vi "REQ Initialize DI.vi"(6 "wait for reply (T)":bool=TRUE, 8 "error in":errorcluster, 10 "Boolean":bool, 11 "DI Channel Setting":T1) -> (0 "error out":errorcluster, 1 "timed out?":bool, 3 "Connect?":bool)   [LabVIEW 2016, in "DAQ Hardware.lvlib"]
doc: "_____\nCreated using DQMH Event Scripter 6.1.0.128."
uses:
  DAQ Hardware.lvlib
  DI Channel Setting.ctl
  REQ Initialize DI Argument--cluster.ctl
  REQ Initialize DI (Reply Payload)--cluster.ctl
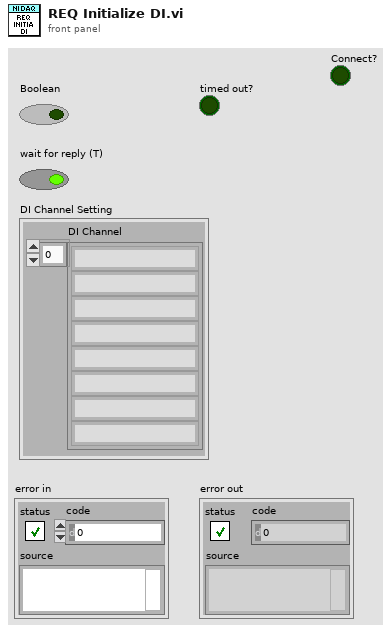
[diagram p1: front panel]
types:
  T1 = typedef "DAQ Hardware.lvlib/DI Channel Setting.ctl" = cluster{"DI Channel":string[]}
  T2 = typedef "DAQ Hardware.lvlib/REQ Initialize DI Argument--cluster.ctl" = cluster{"Boolean":bool, "Wait Notifier":refnum<notifier>, "wait for reply":bool, "DI Channel Setting":T1}
  T3 = typedef "DAQ Hardware.lvlib/Request Events--cluster.ctl" = cluster{"Stop Module":refnum<user-event>, "Show Panel":refnum<user-event>, "Hide Panel":refnum<user-event>, "Get Module Execution Status":refnum<user-event>, "Show Diagram":refnum<user-event>, "REQ Initialize AI":refnum<user-event>, "REQ Initialize AO":refnum<user-event>, "REQ Initialize DI":refnum<user-event>, "REQ Initialize DO":refnum<user-event>, "REQ Write DO":refnum<user-event>, "REQ Acquire AI":refnum<user-event>, "REQ Close Ref":refnum<user-event>, "REQ Write AO":refnum<user-event>, "REQ Update Sample Rate":refnum<user-event>, "REQ Acquire DI":refnum<user-event>, "REQ Wakeup_Helper_loop_AI":refnum<user-event>, "REQ Retry AI":refnum<user-event>, "REQ Wakeup_helper_loop_DI":refnum<user-event>, "REQ Retry DI":refnum<user-event>, "Write AO Data":refnum<user-event>, "REQ Log Data":refnum<user-event>}
  T4 = typedef "DAQ Hardware.lvlib/REQ Initialize DI (Reply Payload)--cluster.ctl" = cluster{"error":errorcluster, "Connect?":bool}
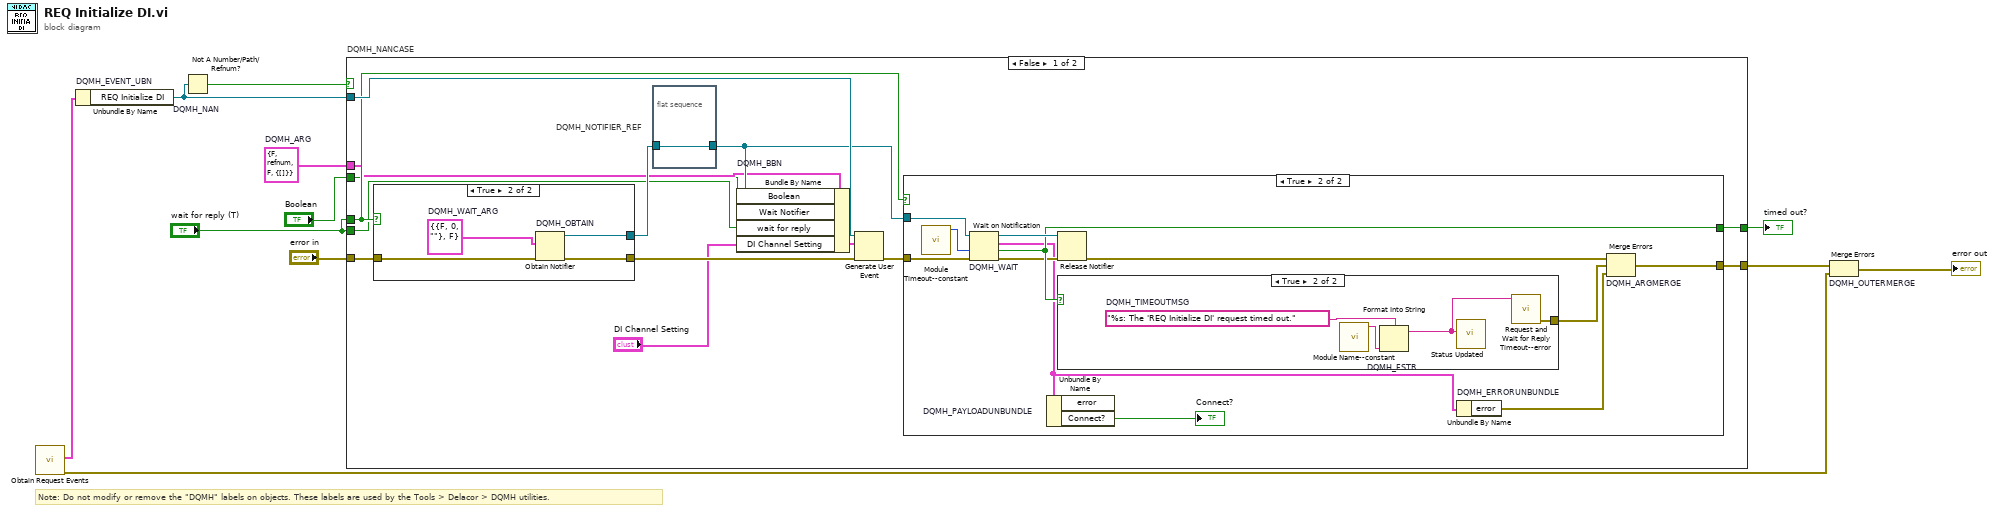
[diagram p0: block diagram]
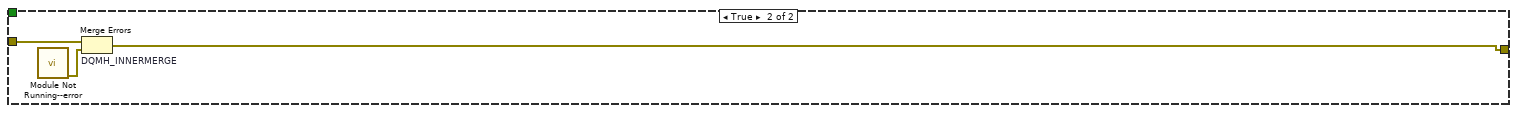
[diagram p5: hidden frame]
diagram:
  w5 = T2 {"Boolean"=FALSE, "Wait Notifier"=refnum, "wait for reply"=FALSE, "DI Channel Setting"={"DI Channel"=[]}}  # DQMH_ARG
  # "Note: Do not modify or remove the \"DQMH\" labels on objects. These labels are used by the Tools > Delacor > DQMH utilities."
  n1 = call "Obtain Request Events.vi"() -> ("error out"=w2:errorcluster, "DAQ Hardware Request Events"=w1:T3)  [unwired: 10 in]
  n2 = Unbundle By Name "DQMH_EVENT_UBN"(w1) -> ("REQ Initialize DI"=w6:refnum<user-event>)
  n3 = Not A Number/Path/Refnum? "DQMH_NAN"(number/path/refnum=w6) -> (NaN/Path/Refnum?=w7:bool)
  n4 = case "DQMH_NANCASE" shown="False" w7 {
    tunnel: "error in" -> [w25 w51]
    tunnel: w6 -> [w23 _]
    tunnel: [w20 w50] -> w8
    tunnel: [w21 _] -> w10
    tunnel: "wait for reply (T)" -> [w18 _]
    tunnel: w5 -> [w15 _]
    tunnel: "Boolean" -> [w14 _]
    tunnel: "wait for reply (T)" -> [w13 _]
    frame False {
      n5 = case shown="True" w18 {
        tunnel: w25 -> [w44 w48]
        tunnel: [w44 w47] -> w22
        tunnel: [_ w45] -> w17
        frame False {
        }
        frame True {
          w46 = T4 {"error"={"status"=FALSE, "code"=0, "source"=""}, "Connect?"=FALSE}  # DQMH_WAIT_ARG
          n6 = Obtain Notifier "DQMH_OBTAIN"(notification data type=w46, error in (no error)=w48) -> (notifier out=w45:refnum<notifier>, error out=w47:errorcluster)  [unwired: 2 in, 1 out]
        }
      }
      n7 = flat-sequence "DQMH_NOTIFIER_REF" {
        tunnel: w17 -> [w26]
        tunnel: [w26] -> w16
        frame #0 {
        }
      }
      n8 = Bundle By Name "DQMH_BBN"(cluster=w15, "Boolean"=w14, "Wait Notifier"=w16, "wait for reply"=w13, "DI Channel Setting"="DI Channel Setting") -> (w19:T2)
      n9 = Generate User Event(user event=w23, event data cluster=w19, error in=w22) -> (error out=w24:errorcluster)  [unwired: 1 in, 1 out]
      n10 = case shown="True" w18 {
        tunnel: w24 -> [w27 w39]
        tunnel: w16 -> [_ w38]
        tunnel: [_ w36] -> w21
        tunnel: [w27 w35] -> w20
        frame False {
        }
        frame True {
          n11 = call "Module Timeout--constant.vi"() -> ("Module Timeout"=w29:i32)  [unwired: 11 in]
          n12 = Wait on Notification "DQMH_WAIT"(notifier=w38, timeout in ms (-1)=w29, error in (no error)=w39) -> (notifier out=w37:refnum<notifier>, notification=w30:T4, timed out?=w36:bool, error out=w34:errorcluster)  [unwired: 1 in]
          n13 = Unbundle By Name "DQMH_PAYLOADUNBUNDLE"(w30) -> ("Connect?"=→"Connect?":bool)  [unwired: 1 out]
          n14 = Release Notifier(notifier=w37, error in (no error)=w34) -> (error out=w33:errorcluster)  [unwired: 1 in, 2 out]
          n15 = case shown="True" w36 {
            tunnel: [_ w41] -> w31
            frame False {
            }
            frame True {
              w43 = "%s: The 'REQ Initialize DI' request timed out."  # DQMH_TIMEOUTMSG
              n16 = call "Module Name--constant.vi"() -> ("Module Name"=w40:string)  [unwired: 11 in]
              n17 = Format Into String "DQMH_FSTR"(format string=w43, w40) -> (resulting string=w42:string)  [unwired: 2 in, 1 out]
              n18 = call "Status Updated.vi"("Status"=w42) -> ()  [unwired: 10 in, 1 out]
              n19 = call "Request and Wait for Reply Timeout--error.vi"("Error Message"=w42) -> ("error out"=w41:errorcluster)  [unwired: 10 in]
            }
          }
          n20 = Unbundle By Name "DQMH_ERRORUNBUNDLE"(w30) -> ("error"=w32:errorcluster)
          n21 = Merge Errors "DQMH_ARGMERGE"(w33, w31, w32) -> (w35:errorcluster)
        }
      }
    }
    frame True {
      n22 = call "Module Not Running--error.vi"() -> ("error out"=w49:errorcluster)  [unwired: 11 in]
      n23 = Merge Errors "DQMH_INNERMERGE"(w51, w49) -> (w50:errorcluster)
    }
  }
  "timed out?" <- w10
  n24 = Merge Errors "DQMH_OUTERMERGE"(w8, w2) -> (→"error out":errorcluster)
